vi "config--display_next and display_previous.vi"(4 "no. of completed_tours":u64 caption="completed_tour currently displayed", 6 "completed_tour currently displayed":u64, 8 "error in (no error)":errorcluster, 10 "display_previous":refnum<vi>, 11 "display_next":refnum<vi>) -> (0 "error out":errorcluster)   [LabVIEW 2020, in "main.lvlib"]
doc: "Blank VI with error handling."
uses:
  main.lvlib
  PTRL/GUI_tools/GUI_tools.lvlib
panel:
  # "Development\ncontrols/indicators useful for development and testing, but which are not outputs of the VI"
  # "Input\nInputs to the VI"
  # "Output\nOutputs of the VI"
  # "Description\n\nBlank VI with error handling case. \n\nSummarize the use of this VI in this space."
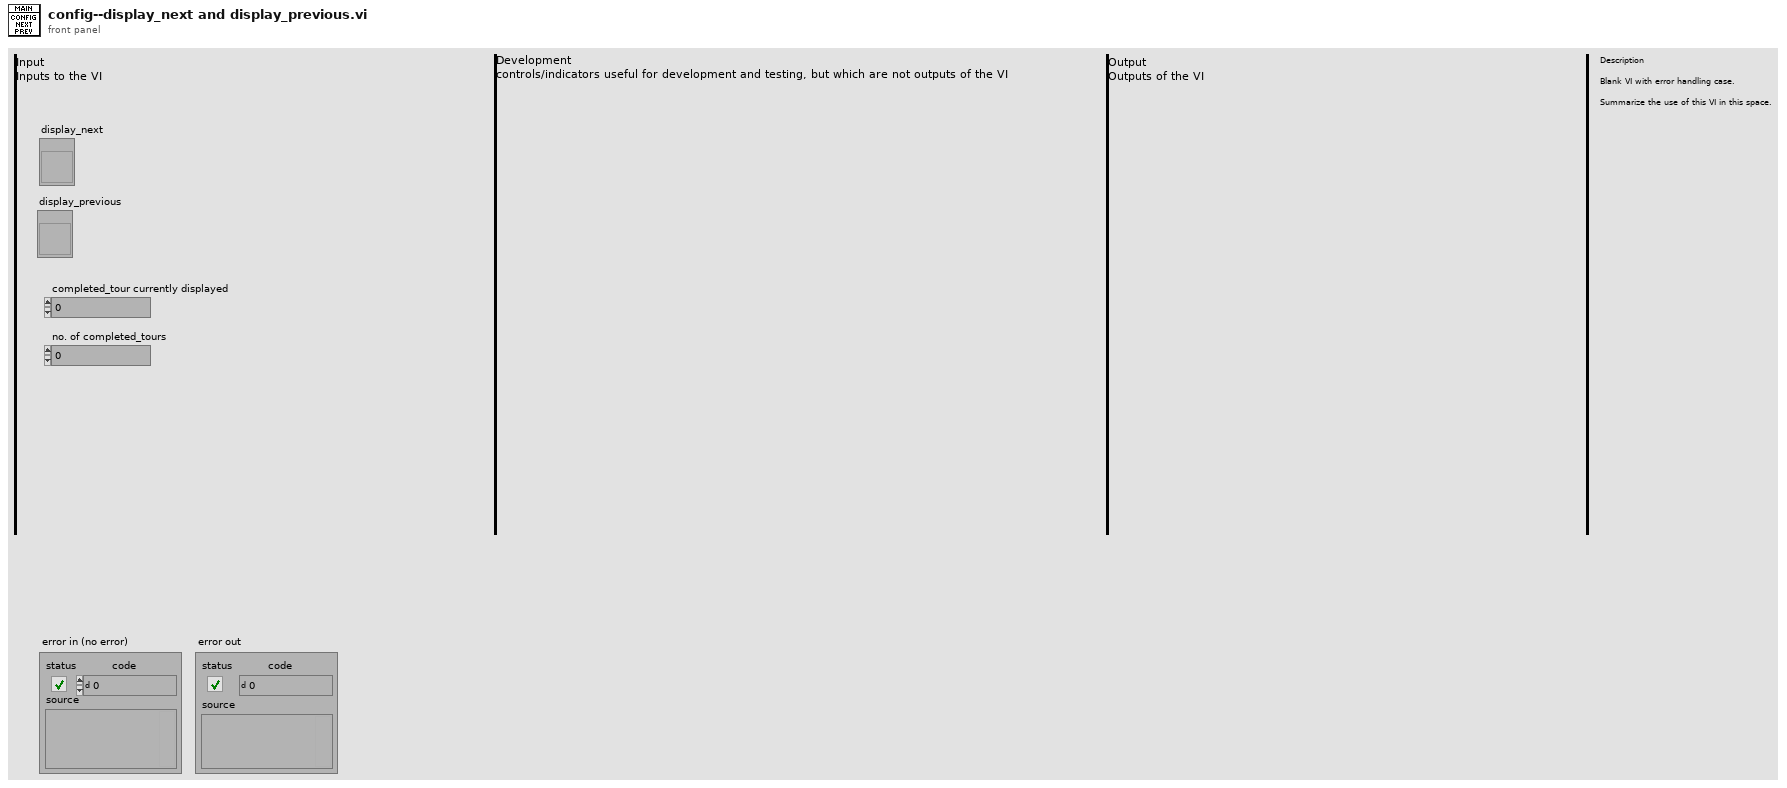
[diagram p1: front panel]
types:
  T1 = enum8{"Enabled", "Disabled", "Disabled and Grayed Out"}
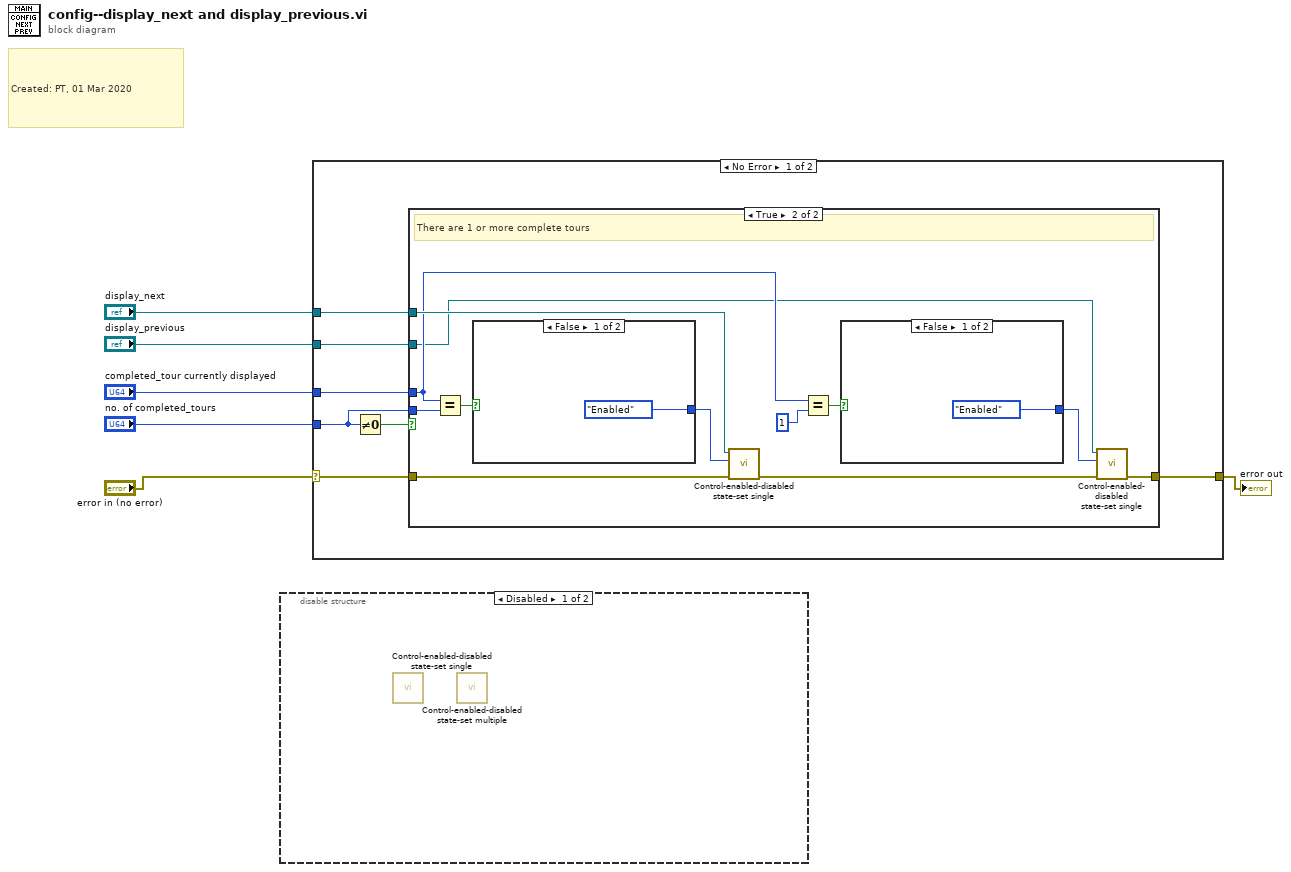
[diagram p0: block diagram]
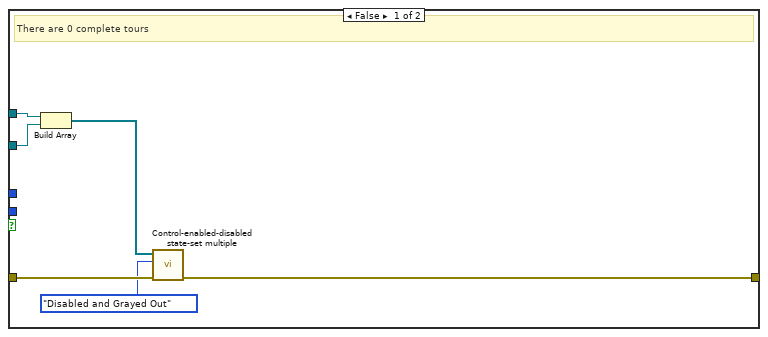
[diagram p2: hidden frame]
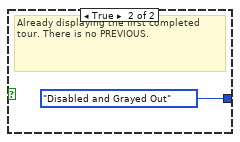
[diagram p3: hidden frame]
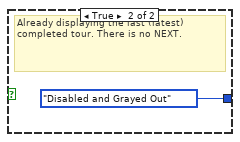
[diagram p4: hidden frame]
diagram:
  # "Created: PT, 01 Mar 2020"
  n1 = disable-structure shown="Disabled" {
    frame Disabled {
      n2 = call "Control-enabled-disabled state-set single.vi"() -> ()  [unwired: 10 in, 2 out]
      n3 = call "Control-enabled-disabled state-set multiple.vi"() -> ()  [unwired: 10 in, 2 out]
    }
    frame Enabled {
    }
  }
  n4 = case shown="No Error" "error in (no error)" {
    selector: "error in (no error)" -> [w13 w36]
    tunnel: [w12 w36] -> w5
    tunnel: "display_next" -> [w10 _]
    tunnel: "display_previous" -> [w9 _]
    tunnel: "no. of completed_tours" -> [w7 _]
    tunnel: "completed_tour currently displayed" -> [w8 _]
    frame No Error {
      n5 = Not Equal To 0?(x=w7) -> (x != 0?=w11:bool)
      n6 = case shown="True" w11 {
        tunnel: w13 -> [w19 w31]
        tunnel: [w18 w20] -> w12
        tunnel: w10 -> [w17 w27]
        tunnel: w9 -> [w16 w21]
        tunnel: w8 -> [_ w23]
        tunnel: w7 -> [_ w30]
        frame False {
          # "There are 0 complete tours"
          n7 = Build Array(w17, w16) -> (w15:refnum<vi>[])
          n8 = call "Control-enabled-disabled state-set multiple.vi"("error in (no error)"=w19, "State"=T1."Disabled and Grayed Out", "Control refs in"=w15) -> ("error out"=w18:errorcluster)  [unwired: 7 in, 1 out]
        }
        frame True {
          # "There are 1 or more complete tours"
          n9 = Equal?(x=w23, y=w30) -> (x = y?=w29:bool)
          n10 = case shown="False" w29 {
            tunnel: [T1."Enabled" ("State") T1."Disabled and Grayed Out" ("State")] -> w28
            frame False {
            }
            frame True {
              # "Already displaying the last (latest) completed tour. There is no NEXT."
            }
          }
          n11 = call "Control-enabled-disabled state-set single.vi"("error in (no error)"=w31, "State"=w28, "Control ref in"=w27) -> ("error out"=w24:errorcluster)  [unwired: 7 in, 1 out]
          n12 = Equal?(x=w23, y=u64 1) -> (x = y?=w25:bool)
          n13 = case shown="False" w25 {
            tunnel: [T1."Enabled" ("State") T1."Disabled and Grayed Out" ("State")] -> w26
            frame False {
            }
            frame True {
              # "Already displaying the first completed tour. There is no PREVIOUS."
            }
          }
          n14 = call "Control-enabled-disabled state-set single.vi"("error in (no error)"=w24, "State"=w26, "Control ref in"=w21) -> ("error out"=w20:errorcluster)  [unwired: 7 in, 1 out]
        }
      }
    }
    frame Error {
    }
  }
  "error out" <- w5
